vi "8_Direct_Time_Tag_Stream_Access.vi"(8 "error in (no error)":errorcluster) -> (0 "error out":errorcluster)   [LabVIEW 2014]
uses:
  SwabianInstruments.TimeTagger
panel:
  in  "Enable evaluation":bool=TRUE
  out "buffer utilization, %":dbl format="%#_3g"
  out "sum of channel numbers":i32
  in  "Nchannels":i32=2 min=1 max=18 step=1
  out "Tag rate":dbl(graph)
  out "hasOverflows":bool
  out "number of time tags":u64
  in  "stop":bool
  in  "Rate divider":i32=4 min=2 step=1
  out "loop iteration":i32
  # "Restart the VI to apply the change"
  # "Can be changed during run-time"
  # "Tag rate  (samples / s) = 50e6 x Nchannels  / Rate divider"
  # "We attempts to aquire the data of the raw time tag stream \nevery 25 ms. Real data readout rate may be limited by CPU."
  # "The number of time tags received should not increase\npermantently otherwise the average data rate is too high \nand the cpu cannot handle the time tag stream which of \ncourse depends highly on the evaluation performed.\n\nBuffer allocation shows how many tags were read \ncompared to the \"n_max_events\" specified \nto the TimeTagStream. When this value reaches 100%, \nit means that we are not reading data fast enough.\nOne can try reducing loop time, increasing buffer size or\noptimizing evaluation algorithm."
  # "Evaluation"
  # "The evaluation done here is useless - but out of each tag \nthe time and channel information is used to calculate something. \nThe complexity of the evaluation method will limit the number of \ntags which can be used. This is defined by CPU processing capability.\n\nExample for a laptop with CPU  i5-7200U @ 2.7GHz:\n Time Tagger 20 - The maximum transfer rate is limited by the USB2 bandwidth to ~8-9 million tags per second\n Time Tagger Ultra - when connected via USB3 one can achieve  ~37 million tags per second and becomes CPU limited."
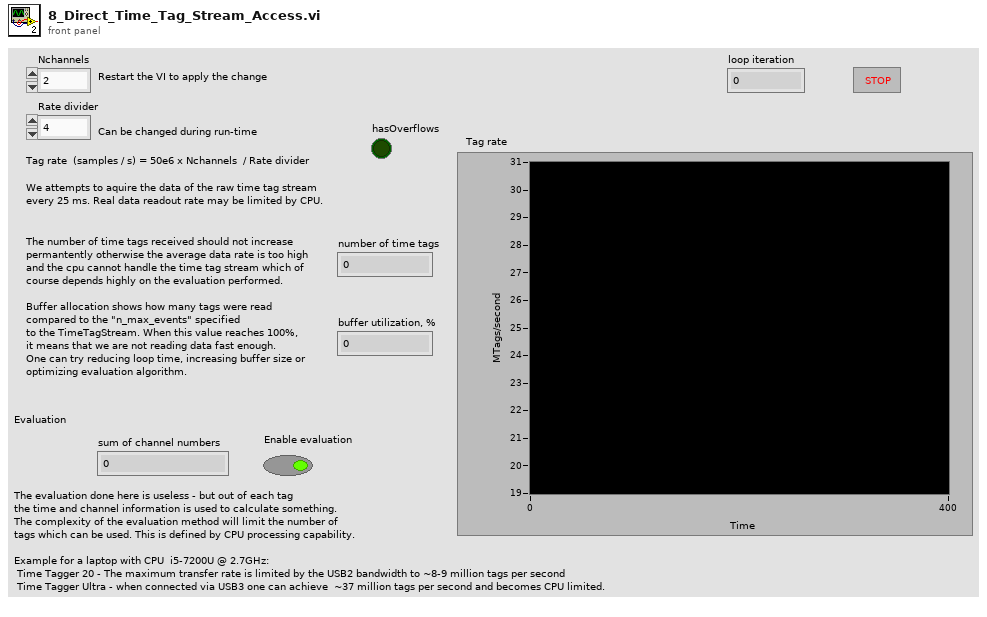
[diagram p1: front panel]
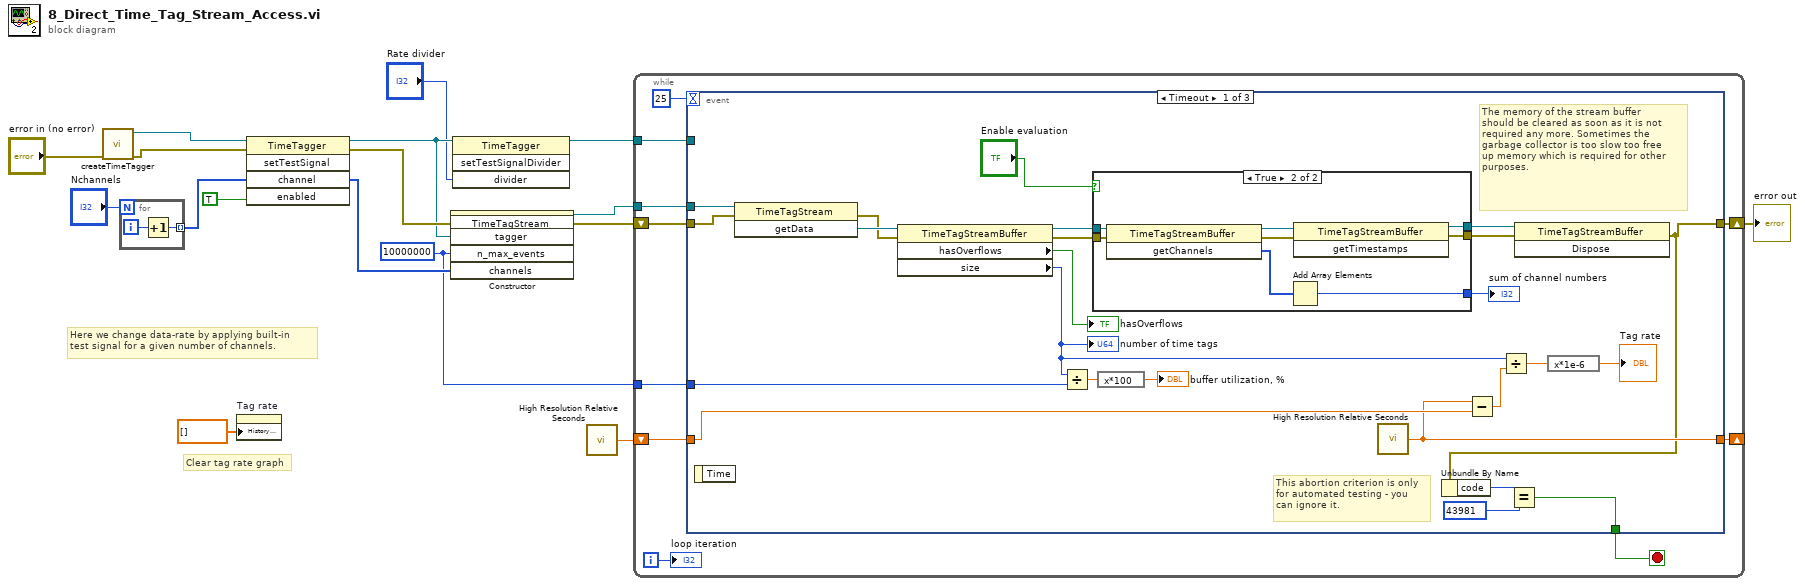
[diagram p0: block diagram]
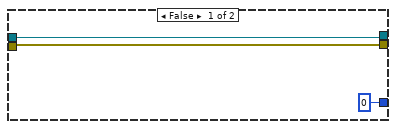
[diagram p2: hidden frame]
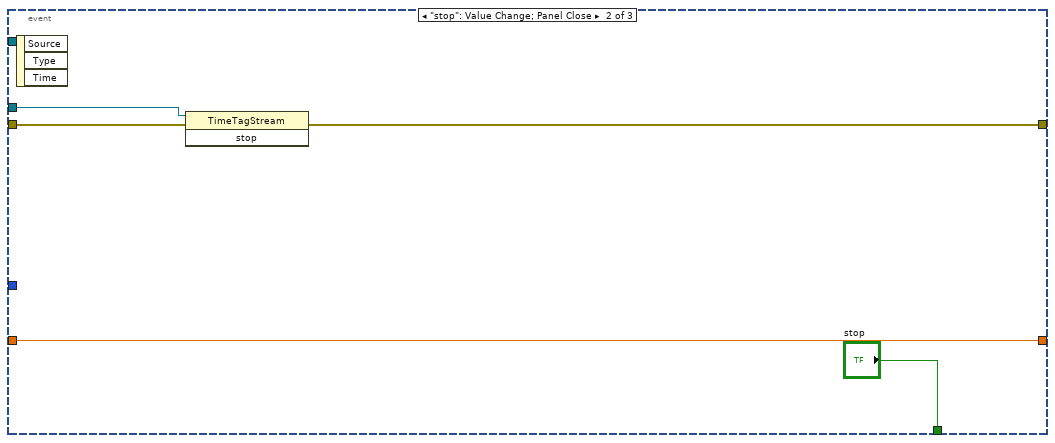
[diagram p3: hidden frame]
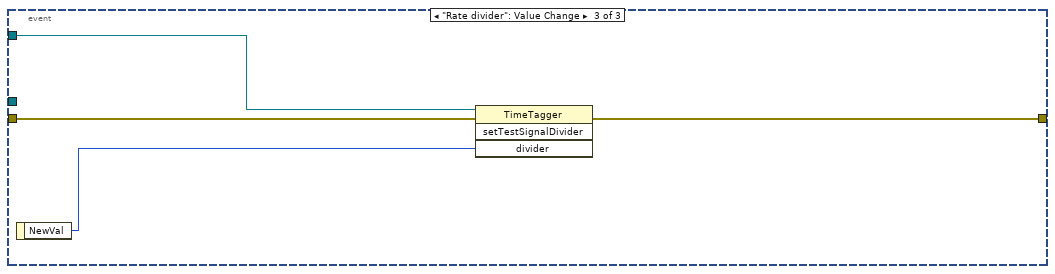
[diagram p4: hidden frame]
diagram:
  w4 = 10000000 ("n_max_events")
  # "Clear tag rate graph"
  # "Here we change data-rate by applying built-in \ntest signal for a given number of channels."
  n1 = call "createTimeTagger.vi"("error in (no error)"="error in (no error)") -> ("error out"=w15:errorcluster, "TimeTagger ref out"=w11:refnum<k24>)  [unwired: 9 in]
  n2 = for {
    N: "Nchannels" -> [_]
    tunnel: [w18] -> w14 mode=indexing
    i -> [w19]
    n3 = Increment(x=w19) -> (x+1=w18:i32)
  }
  n4 = property on="Tag rate" class="WFChart (strict)"("History Data"=dbl[] []) -> ()  [unwired: 2 in, 2 out]
  n5 = invoke class="TimeTagger" method="setTestSignal"(reference=w11, error in=w15, "channel"=w14, "enabled"=TRUE) -> (reference out=w7:refnum<k24>, error out=w16:errorcluster, "channel"=w10:i32[])  [unwired: 1 in, 2 out]
  n6 = constructor class="TimeTagStream"(error in=w16, "tagger"=w7, "n_max_events"=w4, "channels"=w10) -> (reference out=w12:refnum<k24>, error out=w13:errorcluster)  [unwired: 2 in, 4 out]
  n7 = invoke class="TimeTagger" method="setTestSignalDivider"(reference=w7, "divider"="Rate divider") -> (reference out=w5:refnum<k24>)  [unwired: 2 in, 3 out]
  n8 = call <vilib>:"High Resolution Relative Seconds.vi"() -> ("relative seconds"=w9:dbl)
  n9 = while {
    shift-right: [w26] -> w2
    shift-left: w13 -> [w27]
    tunnel: w12 -> [w25]
    tunnel: w5 -> [w23]
    shift-right: [w21] -> _
    shift-left: w9 -> [w22]
    tunnel: w4 -> [w20]
    i -> [w24]
    stop <- w28 stop-if-true
    n10 = event shown="[0] Timeout" {
      selector: _ -> [_ _ _]
      dyn-events: _ -> [_ _ _]
      timeout: 25 -> [_ _ _]
      tunnel: [w30 "stop" _] -> w28
      tunnel: w27 -> [w47 w67 w71]
      tunnel: [w33 w66 w70] -> w26
      tunnel: w25 -> [w48 w68 _]
      tunnel: w23 -> [_ _ w73]
      tunnel: w22 -> [w42 w65 _]
      tunnel: [w41 w65 _] -> w21
      tunnel: w20 -> [w39 _ _]
      event Timeout {
        # "This abortion criterion is only\nfor automated testing - you\ncan ignore it."
        # "The memory of the stream buffer \nshould be cleared as soon as it is not\nrequired any more. Sometimes the\ngarbage collector is too slow too free\nup memory which is required for other\npurposes."
        n11 = event-data() -> ()  [unwired: 1 in, 1 out]
        n12 = invoke class="TimeTagStream" method="getData"(reference=w48, error in=w47) -> (error out=w49:errorcluster, "getData"=w53:refnum<k24>)  [unwired: 1 in, 1 out]
        n13 = property class="TimeTagStreamBuffer"(reference=w53, error in=w49) -> (reference out=w51:refnum<k24>, error out=w50:errorcluster, "hasOverflows"=→"hasOverflows":bool, "size"=w40:u64)
        "number of time tags" <- w40
        n14 = Divide(x=w40, y=w39) -> (x/y=w38:dbl)
        n15 = case shown="True" "Enable evaluation" {
          tunnel: w51 -> [w56 w64]
          tunnel: w50 -> [w55 w63]
          tunnel: [w55 w62] -> w46
          tunnel: [w56 w61] -> w45
          tunnel: [0 w57] -> w35
          frame False {
          }
          frame True {
            n16 = invoke class="TimeTagStreamBuffer" method="getChannels"(reference=w64, error in=w63) -> (reference out=w60:refnum<k24>, error out=w59:errorcluster, "getChannels"=w58:i32[])  [unwired: 1 in]
            n17 = Add Array Elements(numeric array=w58) -> (sum=w57:i32)
            n18 = invoke class="TimeTagStreamBuffer" method="getTimestamps"(reference=w60, error in=w59) -> (reference out=w61:refnum<k24>, error out=w62:errorcluster)  [unwired: 1 in, 1 out]
          }
        }
        "sum of channel numbers" <- w35
        n19 = expression code="x*100"(w38) -> (→"buffer utilization, %":dbl)
        n20 = call <vilib>:"High Resolution Relative Seconds.vi"() -> ("relative seconds"=w41:dbl)
        n21 = Subtract(x=w41, y=w42) -> (x-y=w43:dbl)
        n22 = Divide(x=w40, y=w43) -> (x/y=w44:dbl)
        n23 = invoke class="TimeTagStreamBuffer" method="Dispose"(reference=w45, error in=w46) -> (error out=w33:errorcluster)  [unwired: 1 in, 2 out]
        n24 = Unbundle By Name(w33) -> ("code"=w32:i32)
        n25 = Equal?(x=w32, y=43981) -> (x = y?=w30:bool)
        n26 = expression code="x*1e-6"(w44) -> (→"Tag rate":dbl)
      }
      event "stop": Value Change; Panel Close {
        n27 = event-data() -> ()  [unwired: 1 in, 3 out]
        n28 = invoke class="TimeTagStream" method="stop"(reference=w68, error in=w67) -> (error out=w66:errorcluster)  [unwired: 1 in, 2 out]
      }
      event "Rate divider": Value Change {
        n29 = event-data() -> ("NewVal"=w72:i32)  [unwired: 1 in]
        n30 = invoke class="TimeTagger" method="setTestSignalDivider"(reference=w73, error in=w71, "divider"=w72) -> (error out=w70:errorcluster)  [unwired: 1 in, 3 out]
      }
    }
    "loop iteration" <- w24
  }
  "error out" <- w2
